vi "remove tag from dictionary.vi"(8 "error in":errorcluster, 10 "system tag":refnum<class "tag descriptor.lvclass">, 11 "data dictionary in":refnum<class "data dictionary.lvclass">) -> (0 "error out":errorcluster, 3 "data dictionary out":refnum<class "data dictionary.lvclass">)   [LabVIEW 2013, in "tag bus.lvlib" / "data dictionary.lvclass"]
doc: "Removes a tag from the data dictionary. This function uses the name and data type fields of the descriptor."
uses:
  data dictionary.lvclass
  tag/tag descriptor.lvclass
  tag/tag descriptor.lvclass/tag descriptor.ctl
  data dictionary.lvclass/data dictionary.ctl
  search/binary search.lvlib
  tag bus.lvlib
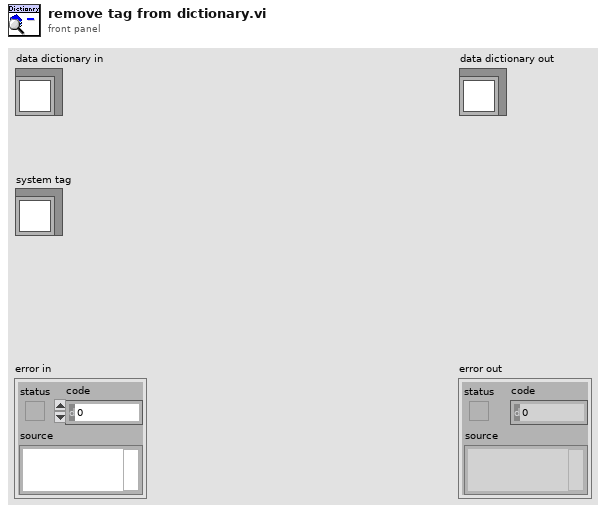
[diagram p1: front panel]
types:
  T1 = typedef "tag bus.lvlib/tag descriptor.lvclass/Data Type.ctl" = enum16{"Double", "Single", "I64", "I32", "I16", "I8", "U64", "U32", "U16", "U8", "Boolean", "String", "Array of Double", "Array of Single", "Array of I64", "Array of I32", "Array of I16", "Array of I8", "Array of U64", "Array of U32", "Array of U16", "Array of U8", "Array of Boolean", "Array of String"}
  T2 = typedef "tag bus.lvlib/binary search.lvlib/sorted list.ctl" = cluster{"sorted strings":string[], "sorted indices":i32[]}
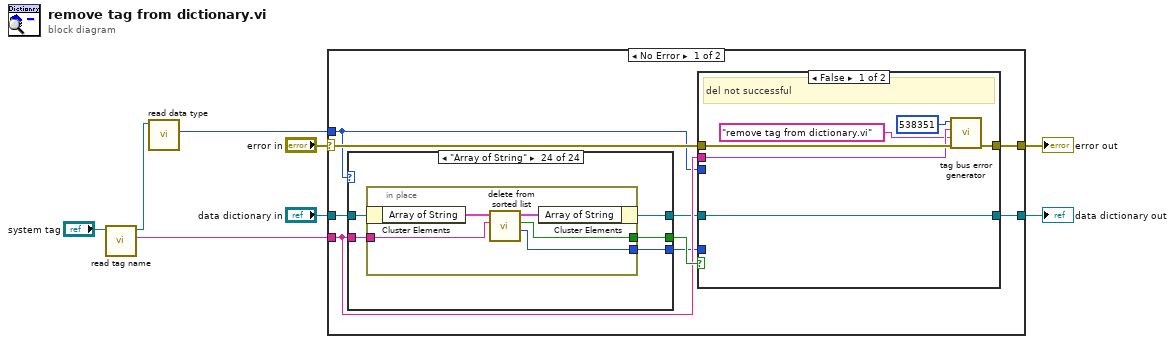
[diagram p0: block diagram]
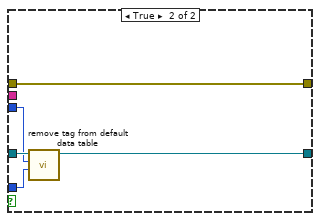
[diagram p2: hidden frame]
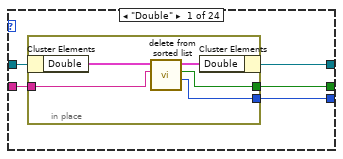
[diagram p3: hidden frame]
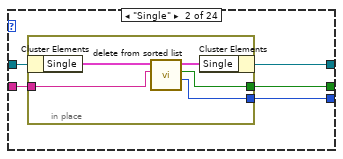
[diagram p4: hidden frame]
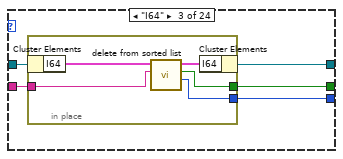
[diagram p5: hidden frame]
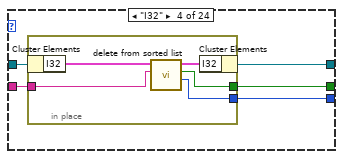
[diagram p6: hidden frame]
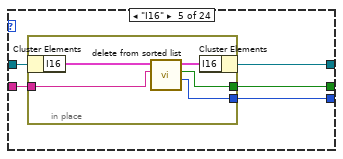
[diagram p7: hidden frame]
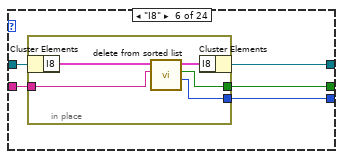
[diagram p8: hidden frame]
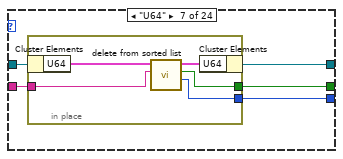
[diagram p9: hidden frame]
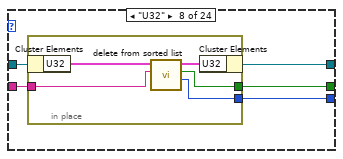
[diagram p10: hidden frame]
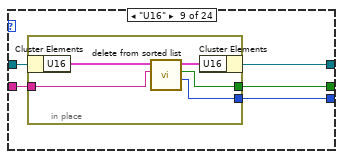
[diagram p11: hidden frame]
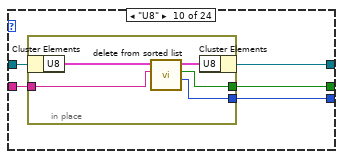
[diagram p12: hidden frame]
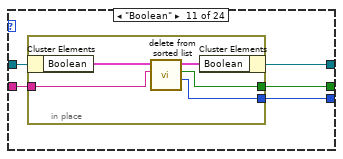
[diagram p13: hidden frame]
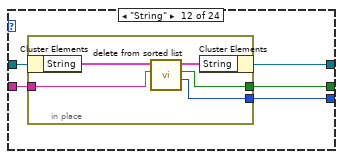
[diagram p14: hidden frame]
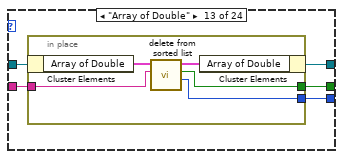
[diagram p15: hidden frame]
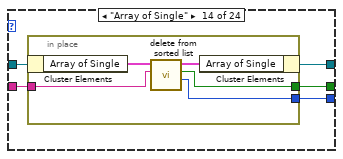
[diagram p16: hidden frame]
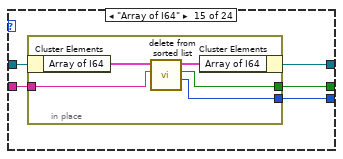
[diagram p17: hidden frame]
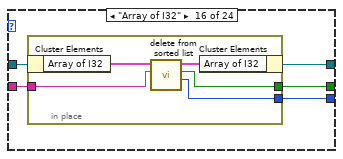
[diagram p18: hidden frame]
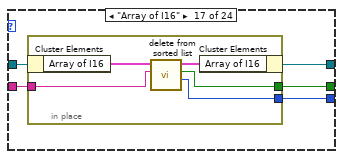
[diagram p19: hidden frame]
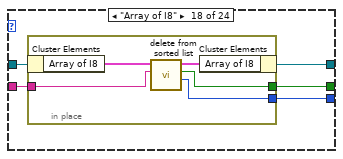
[diagram p20: hidden frame]
diagram:
  n1 = call "read tag name.vi"("system tag in"="system tag") -> ("name"=w5:string, "system tag out"=w3:refnum<class "tag descriptor.lvclass">)  [unwired: 8 in, 1 out]
  n2 = call "read data type.vi"("system tag in"=w3) -> ("data type"=w4:T1)  [unwired: 8 in, 2 out]
  n3 = case shown="No Error" "error in" {
    selector: "error in" -> [w13 w270]
    tunnel: [w17 w270] -> w8
    tunnel: [w12 w269] -> w7
    tunnel: w5 -> [w15 _]
    tunnel: w4 -> [w10 _]
    tunnel: "data dictionary in" -> [w14 w269]
    frame No Error {
      n4 = case shown="\"Array of String\"" w10 {
        tunnel: w14 -> [w33 w43 w53 w63 w73 w83 w93 w103 w113 w123 w133 w143 w153 w163 w173 w183 w193 w203 w213 w223 w233 w243 w253 w263]
        tunnel: [w32 w42 w52 w62 w72 w82 w92 w102 w112 w122 w132 w142 w152 w162 w172 w182 w192 w202 w212 w222 w232 w242 w252 w262] -> w11
        tunnel: w15 -> [w31 w41 w51 w61 w71 w81 w91 w101 w111 w121 w131 w141 w151 w161 w171 w181 w191 w201 w211 w221 w231 w241 w251 w261]
        tunnel: [w30 w40 w50 w60 w70 w80 w90 w100 w110 w120 w130 w140 w150 w160 w170 w180 w190 w200 w210 w220 w230 w240 w250 w260] -> w16
        tunnel: [w29 w39 w49 w59 w69 w79 w89 w99 w109 w119 w129 w139 w149 w159 w169 w179 w189 w199 w209 w219 w229 w239 w249 w259] -> w9
        frame "Double" {
          n5 = in-place {
            in-place-border: w31 -> [w35]
            in-place-border: [w38] -> w30
            in-place-border: [w34] -> w29
            n6 = in-place-cluster #1(w33) -> ("Double"=w36:T2)
            n7 = call "delete from sorted list.vi"("element to delete"=w35, "sorted list in"=w36) -> ("deleted index"=w34:i32, "success?"=w38:bool, "sorted list out"=w37:T2)  [unwired: 7 in]
            n8 = in-place-cluster #1("Double"=w37) -> (w32:refnum<class "data dictionary.lvclass">)
          }
        }
        frame "Single" {
          n9 = in-place {
            in-place-border: w41 -> [w45]
            in-place-border: [w48] -> w40
            in-place-border: [w44] -> w39
            n10 = in-place-cluster #2(w43) -> ("Single"=w46:T2)
            n11 = call "delete from sorted list.vi"("element to delete"=w45, "sorted list in"=w46) -> ("deleted index"=w44:i32, "success?"=w48:bool, "sorted list out"=w47:T2)  [unwired: 7 in]
            n12 = in-place-cluster #2("Single"=w47) -> (w42:refnum<class "data dictionary.lvclass">)
          }
        }
        frame "I64" {
          n13 = in-place {
            in-place-border: w51 -> [w55]
            in-place-border: [w58] -> w50
            in-place-border: [w54] -> w49
            n14 = in-place-cluster #3(w53) -> ("I64"=w56:T2)
            n15 = call "delete from sorted list.vi"("element to delete"=w55, "sorted list in"=w56) -> ("deleted index"=w54:i32, "success?"=w58:bool, "sorted list out"=w57:T2)  [unwired: 7 in]
            n16 = in-place-cluster #3("I64"=w57) -> (w52:refnum<class "data dictionary.lvclass">)
          }
        }
        frame "I32" {
          n17 = in-place {
            in-place-border: w61 -> [w65]
            in-place-border: [w68] -> w60
            in-place-border: [w64] -> w59
            n18 = in-place-cluster #4(w63) -> ("I32"=w66:T2)
            n19 = call "delete from sorted list.vi"("element to delete"=w65, "sorted list in"=w66) -> ("deleted index"=w64:i32, "success?"=w68:bool, "sorted list out"=w67:T2)  [unwired: 7 in]
            n20 = in-place-cluster #4("I32"=w67) -> (w62:refnum<class "data dictionary.lvclass">)
          }
        }
        frame "I16" {
          n21 = in-place {
            in-place-border: w71 -> [w75]
            in-place-border: [w78] -> w70
            in-place-border: [w74] -> w69
            n22 = in-place-cluster #5(w73) -> ("I16"=w76:T2)
            n23 = call "delete from sorted list.vi"("element to delete"=w75, "sorted list in"=w76) -> ("deleted index"=w74:i32, "success?"=w78:bool, "sorted list out"=w77:T2)  [unwired: 7 in]
            n24 = in-place-cluster #5("I16"=w77) -> (w72:refnum<class "data dictionary.lvclass">)
          }
        }
        frame "I8" {
          n25 = in-place {
            in-place-border: w81 -> [w85]
            in-place-border: [w88] -> w80
            in-place-border: [w84] -> w79
            n26 = in-place-cluster #6(w83) -> ("I8"=w86:T2)
            n27 = call "delete from sorted list.vi"("element to delete"=w85, "sorted list in"=w86) -> ("deleted index"=w84:i32, "success?"=w88:bool, "sorted list out"=w87:T2)  [unwired: 7 in]
            n28 = in-place-cluster #6("I8"=w87) -> (w82:refnum<class "data dictionary.lvclass">)
          }
        }
        frame "U64" {
          n29 = in-place {
            in-place-border: w91 -> [w95]
            in-place-border: [w98] -> w90
            in-place-border: [w94] -> w89
            n30 = in-place-cluster #7(w93) -> ("U64"=w96:T2)
            n31 = call "delete from sorted list.vi"("element to delete"=w95, "sorted list in"=w96) -> ("deleted index"=w94:i32, "success?"=w98:bool, "sorted list out"=w97:T2)  [unwired: 7 in]
            n32 = in-place-cluster #7("U64"=w97) -> (w92:refnum<class "data dictionary.lvclass">)
          }
        }
        frame "U32" {
          n33 = in-place {
            in-place-border: w101 -> [w105]
            in-place-border: [w108] -> w100
            in-place-border: [w104] -> w99
            n34 = in-place-cluster #8(w103) -> ("U32"=w106:T2)
            n35 = call "delete from sorted list.vi"("element to delete"=w105, "sorted list in"=w106) -> ("deleted index"=w104:i32, "success?"=w108:bool, "sorted list out"=w107:T2)  [unwired: 7 in]
            n36 = in-place-cluster #8("U32"=w107) -> (w102:refnum<class "data dictionary.lvclass">)
          }
        }
        frame "U16" {
          n37 = in-place {
            in-place-border: w111 -> [w115]
            in-place-border: [w118] -> w110
            in-place-border: [w114] -> w109
            n38 = in-place-cluster #9(w113) -> ("U16"=w116:T2)
            n39 = call "delete from sorted list.vi"("element to delete"=w115, "sorted list in"=w116) -> ("deleted index"=w114:i32, "success?"=w118:bool, "sorted list out"=w117:T2)  [unwired: 7 in]
            n40 = in-place-cluster #9("U16"=w117) -> (w112:refnum<class "data dictionary.lvclass">)
          }
        }
        frame "U8" {
          n41 = in-place {
            in-place-border: w121 -> [w125]
            in-place-border: [w128] -> w120
            in-place-border: [w124] -> w119
            n42 = in-place-cluster #10(w123) -> ("U8"=w126:T2)
            n43 = call "delete from sorted list.vi"("element to delete"=w125, "sorted list in"=w126) -> ("deleted index"=w124:i32, "success?"=w128:bool, "sorted list out"=w127:T2)  [unwired: 7 in]
            n44 = in-place-cluster #10("U8"=w127) -> (w122:refnum<class "data dictionary.lvclass">)
          }
        }
        frame "Boolean" {
          n45 = in-place {
            in-place-border: w131 -> [w135]
            in-place-border: [w138] -> w130
            in-place-border: [w134] -> w129
            n46 = in-place-cluster #11(w133) -> ("Boolean"=w136:T2)
            n47 = call "delete from sorted list.vi"("element to delete"=w135, "sorted list in"=w136) -> ("deleted index"=w134:i32, "success?"=w138:bool, "sorted list out"=w137:T2)  [unwired: 7 in]
            n48 = in-place-cluster #11("Boolean"=w137) -> (w132:refnum<class "data dictionary.lvclass">)
          }
        }
        frame "String" {
          n49 = in-place {
            in-place-border: w141 -> [w145]
            in-place-border: [w148] -> w140
            in-place-border: [w144] -> w139
            n50 = in-place-cluster #12(w143) -> ("String"=w146:T2)
            n51 = call "delete from sorted list.vi"("element to delete"=w145, "sorted list in"=w146) -> ("deleted index"=w144:i32, "success?"=w148:bool, "sorted list out"=w147:T2)  [unwired: 7 in]
            n52 = in-place-cluster #12("String"=w147) -> (w142:refnum<class "data dictionary.lvclass">)
          }
        }
        frame "Array of Double" {
          n53 = in-place {
            in-place-border: w151 -> [w155]
            in-place-border: [w158] -> w150
            in-place-border: [w154] -> w149
            n54 = in-place-cluster #13(w153) -> ("Array of Double"=w156:T2)
            n55 = call "delete from sorted list.vi"("element to delete"=w155, "sorted list in"=w156) -> ("deleted index"=w154:i32, "success?"=w158:bool, "sorted list out"=w157:T2)  [unwired: 7 in]
            n56 = in-place-cluster #13("Array of Double"=w157) -> (w152:refnum<class "data dictionary.lvclass">)
          }
        }
        frame "Array of Single" {
          n57 = in-place {
            in-place-border: w161 -> [w165]
            in-place-border: [w168] -> w160
            in-place-border: [w164] -> w159
            n58 = in-place-cluster #14(w163) -> ("Array of Single"=w166:T2)
            n59 = call "delete from sorted list.vi"("element to delete"=w165, "sorted list in"=w166) -> ("deleted index"=w164:i32, "success?"=w168:bool, "sorted list out"=w167:T2)  [unwired: 7 in]
            n60 = in-place-cluster #14("Array of Single"=w167) -> (w162:refnum<class "data dictionary.lvclass">)
          }
        }
        frame "Array of I64" {
          n61 = in-place {
            in-place-border: w171 -> [w175]
            in-place-border: [w178] -> w170
            in-place-border: [w174] -> w169
            n62 = in-place-cluster #15(w173) -> ("Array of I64"=w176:T2)
            n63 = call "delete from sorted list.vi"("element to delete"=w175, "sorted list in"=w176) -> ("deleted index"=w174:i32, "success?"=w178:bool, "sorted list out"=w177:T2)  [unwired: 7 in]
            n64 = in-place-cluster #15("Array of I64"=w177) -> (w172:refnum<class "data dictionary.lvclass">)
          }
        }
        frame "Array of I32" {
          n65 = in-place {
            in-place-border: w181 -> [w185]
            in-place-border: [w188] -> w180
            in-place-border: [w184] -> w179
            n66 = in-place-cluster #16(w183) -> ("Array of I32"=w186:T2)
            n67 = call "delete from sorted list.vi"("element to delete"=w185, "sorted list in"=w186) -> ("deleted index"=w184:i32, "success?"=w188:bool, "sorted list out"=w187:T2)  [unwired: 7 in]
            n68 = in-place-cluster #16("Array of I32"=w187) -> (w182:refnum<class "data dictionary.lvclass">)
          }
        }
        frame "Array of I16" {
          n69 = in-place {
            in-place-border: w191 -> [w195]
            in-place-border: [w198] -> w190
            in-place-border: [w194] -> w189
            n70 = in-place-cluster #17(w193) -> ("Array of I16"=w196:T2)
            n71 = call "delete from sorted list.vi"("element to delete"=w195, "sorted list in"=w196) -> ("deleted index"=w194:i32, "success?"=w198:bool, "sorted list out"=w197:T2)  [unwired: 7 in]
            n72 = in-place-cluster #17("Array of I16"=w197) -> (w192:refnum<class "data dictionary.lvclass">)
          }
        }
        frame "Array of I8" {
          n73 = in-place {
            in-place-border: w201 -> [w205]
            in-place-border: [w208] -> w200
            in-place-border: [w204] -> w199
            n74 = in-place-cluster #18(w203) -> ("Array of I8"=w206:T2)
            n75 = call "delete from sorted list.vi"("element to delete"=w205, "sorted list in"=w206) -> ("deleted index"=w204:i32, "success?"=w208:bool, "sorted list out"=w207:T2)  [unwired: 7 in]
            n76 = in-place-cluster #18("Array of I8"=w207) -> (w202:refnum<class "data dictionary.lvclass">)
          }
        }
        frame "Array of U64" {
          n77 = in-place {
            in-place-border: w211 -> [w215]
            in-place-border: [w218] -> w210
            in-place-border: [w214] -> w209
            n78 = in-place-cluster #19(w213) -> ("Array of U64"=w216:T2)
            n79 = call "delete from sorted list.vi"("element to delete"=w215, "sorted list in"=w216) -> ("deleted index"=w214:i32, "success?"=w218:bool, "sorted list out"=w217:T2)  [unwired: 7 in]
            n80 = in-place-cluster #19("Array of U64"=w217) -> (w212:refnum<class "data dictionary.lvclass">)
          }
        }
        frame "Array of U32" {
          n81 = in-place {
            in-place-border: w221 -> [w225]
            in-place-border: [w228] -> w220
            in-place-border: [w224] -> w219
            n82 = in-place-cluster #20(w223) -> ("Array of U32"=w226:T2)
            n83 = call "delete from sorted list.vi"("element to delete"=w225, "sorted list in"=w226) -> ("deleted index"=w224:i32, "success?"=w228:bool, "sorted list out"=w227:T2)  [unwired: 7 in]
            n84 = in-place-cluster #20("Array of U32"=w227) -> (w222:refnum<class "data dictionary.lvclass">)
          }
        }
        frame "Array of U16" {
          n85 = in-place {
            in-place-border: w231 -> [w235]
            in-place-border: [w238] -> w230
            in-place-border: [w234] -> w229
            n86 = in-place-cluster #21(w233) -> ("Array of U16"=w236:T2)
            n87 = call "delete from sorted list.vi"("element to delete"=w235, "sorted list in"=w236) -> ("deleted index"=w234:i32, "success?"=w238:bool, "sorted list out"=w237:T2)  [unwired: 7 in]
            n88 = in-place-cluster #21("Array of U16"=w237) -> (w232:refnum<class "data dictionary.lvclass">)
          }
        }
        frame "Array of U8" {
          n89 = in-place {
            in-place-border: w241 -> [w245]
            in-place-border: [w248] -> w240
            in-place-border: [w244] -> w239
            n90 = in-place-cluster #22(w243) -> ("Array of U8"=w246:T2)
            n91 = call "delete from sorted list.vi"("element to delete"=w245, "sorted list in"=w246) -> ("deleted index"=w244:i32, "success?"=w248:bool, "sorted list out"=w247:T2)  [unwired: 7 in]
            n92 = in-place-cluster #22("Array of U8"=w247) -> (w242:refnum<class "data dictionary.lvclass">)
          }
        }
        frame "Array of Boolean" {
          n93 = in-place {
            in-place-border: w251 -> [w255]
            in-place-border: [w258] -> w250
            in-place-border: [w254] -> w249
            n94 = in-place-cluster #23(w253) -> ("Array of Boolean"=w256:T2)
            n95 = call "delete from sorted list.vi"("element to delete"=w255, "sorted list in"=w256) -> ("deleted index"=w254:i32, "success?"=w258:bool, "sorted list out"=w257:T2)  [unwired: 7 in]
            n96 = in-place-cluster #23("Array of Boolean"=w257) -> (w252:refnum<class "data dictionary.lvclass">)
          }
        }
        frame "Array of String" {
          n97 = in-place {
            in-place-border: w261 -> [w265]
            in-place-border: [w268] -> w260
            in-place-border: [w264] -> w259
            n98 = in-place-cluster #24(w263) -> ("Array of String"=w266:T2)
            n99 = call "delete from sorted list.vi"("element to delete"=w265, "sorted list in"=w266) -> ("deleted index"=w264:i32, "success?"=w268:bool, "sorted list out"=w267:T2)  [unwired: 7 in]
            n100 = in-place-cluster #24("Array of String"=w267) -> (w262:refnum<class "data dictionary.lvclass">)
          }
        }
      }
      n101 = case shown="False" w16 {
        tunnel: w13 -> [w23 w26]
        tunnel: [w22 w26] -> w17
        tunnel: w15 -> [w20 _]
        tunnel: [w19 w28] -> w12
        tunnel: w11 -> [w19 w27]
        tunnel: w10 -> [_ w25]
        tunnel: w9 -> [_ w24]
        frame False {
          # "del not successful"
          n102 = call "tag bus error generator.vi"("error in"=w23, "source"="remove tag from dictionary.vi", "append error message"=w20, "error code (0)"=538351) -> ("error out"=w22:errorcluster)  [unwired: 5 in]
        }
        frame True {
          n103 = call "remove tag from default data table.vi"("index"=w24, "data type"=w25, "data dictionary in"=w27) -> ("data dictionary out"=w28:refnum<class "data dictionary.lvclass">)  [unwired: 8 in]
        }
      }
    }
    frame Error {
    }
  }
  "error out" <- w8
  "data dictionary out" <- w7
